vi "Stop_PulseBlaster.vi"(1 "path in":path=path "C:/SpinCore/SpinAPI/lib/spinapi64.dll") -> (0 "path out":path)   [LabVIEW 2015]
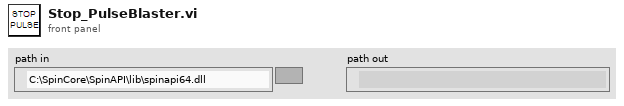
[diagram p1: front panel]
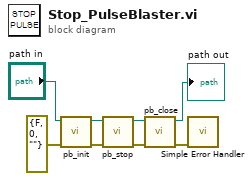
[diagram p0: block diagram]
diagram:
  n1 = call "pb_init.vi"("error in (no error)"=errorcluster {"status"=FALSE, "code"=0, "source"=""}, "path in"="path in") -> ("error out"=w4:errorcluster, "path out"=w8:path)  [unwired: 8 in]
  n2 = call "pb_stop.vi"("error in (no error)"=w4, "path in"=w8) -> ("error out"=w3:errorcluster, "path out"=w7:path)  [unwired: 8 in]
  n3 = call "pb_close.vi"("error in (no error)"=w3, "path in"=w7) -> ("error out"=w2:errorcluster, "path out"=→"path out":path)  [unwired: 8 in]
  n4 = call <vilib>:"Simple Error Handler.vi"("error in (no error)"=w2) -> ()  [unwired: 4 in, 5 out]
